vi "PLCpolling.vi"(8 "error in":errorcluster, 10 "PLC cluster":T1) -> (0 "error out":errorcluster, 1 "172.18.214.225":string[](array[string]), 2 "172.18.214.231":string[](array[string]))   [LabVIEW 2014]
uses:
  PLC-libnodave/PLC_Libnodave_wrapper_areaType.ctl
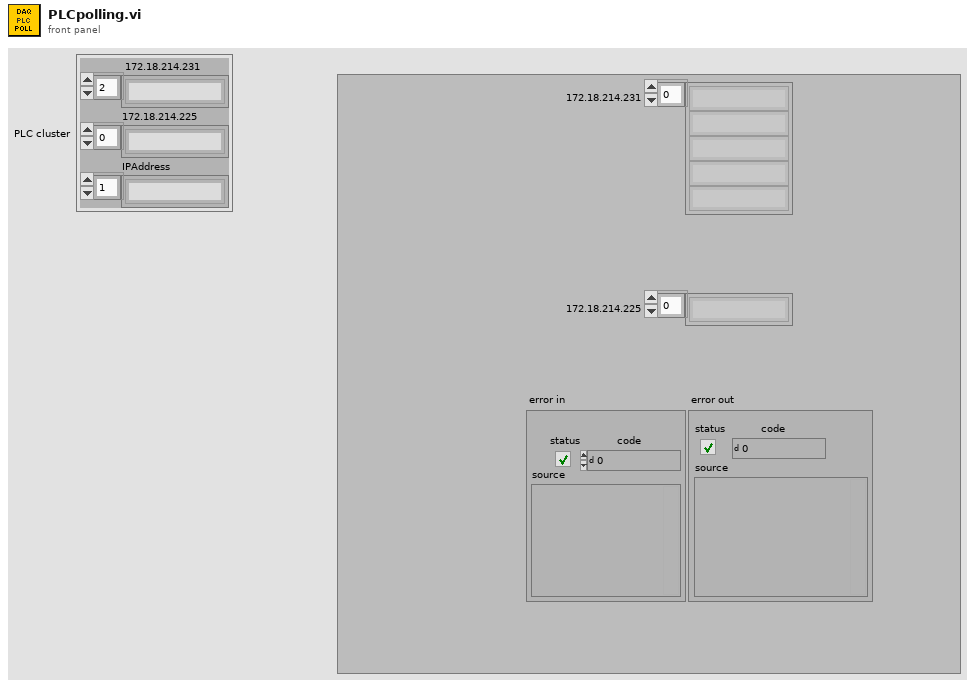
[diagram p1: front panel]
types:
  T1 = cluster{" 172.18.214.231":string[], "172.18.214.225":string[], "IPAddress":string[]}
  T2 = typedef "PLC_Libnodave_wrapper_areaType.ctl" = i32
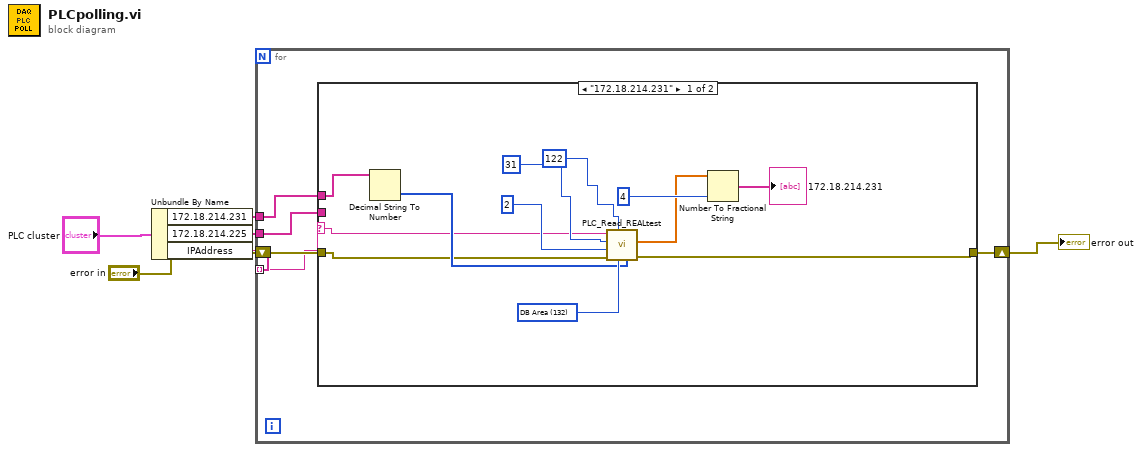
[diagram p0: block diagram]
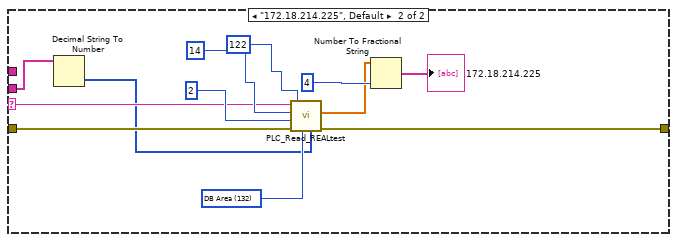
[diagram p2: hidden frame]
diagram:
  n1 = Unbundle By Name("PLC cluster") -> ("172.18.214.231"=w2:string[], "172.18.214.225"=w1:string[], "IPAddress"=w3:string[])
  n2 = for {
    shift-right: [w10] -> w5
    shift-left: "error in" -> [w11]
    tunnel: w3 -> [w9] mode=indexing
    tunnel: w2 -> [w8]
    tunnel: w1 -> [w7]
    n3 = case shown="\"172.18.214.231\"" w9 {
      selector: w9 -> [w16 w28]
      tunnel: w11 -> [w15 w31]
      tunnel: [w17 w32] -> w10
      tunnel: w8 -> [w12 _]
      tunnel: w7 -> [_ w24]
      frame "172.18.214.231" {
        w20 = T2 132 items=["P Area"=128, "I Area"=129, "O Area"=130, "M Area"=131, "DB Area"=132, "Counter Area"=40, "Timer Area"=41] ("areaType")
        n4 = Decimal String To Number(string=w12) -> (number=w18:i32[])  [unwired: 2 in, 1 out]
        n5 = call "PLC_Read_REALtest.vi"("addresses"=w18, "areaType"=w20, "cpProtocol"=122, "Error In"=w15, "slot"=2, "dataBlock"=31, "ip"=w16) -> ("Error Out"=w17:errorcluster, "results"=w14:dbl[])  [unwired: 3 in]
        n6 = Number To Fractional String(number=w14, precision (6)=i16 4) -> (F-format string=→"172.18.214.231":string[])  [unwired: 2 in]
      }
      frame "172.18.214.225", Default {
        w30 = T2 132 items=["P Area"=128, "I Area"=129, "O Area"=130, "M Area"=131, "DB Area"=132, "Counter Area"=40, "Timer Area"=41] ("areaType")
        n7 = Decimal String To Number(string=w24) -> (number=w27:i32[])  [unwired: 2 in, 1 out]
        n8 = call "PLC_Read_REALtest.vi"("addresses"=w27, "areaType"=w30, "cpProtocol"=122, "Error In"=w31, "slot"=2, "dataBlock"=14, "ip"=w28) -> ("Error Out"=w32:errorcluster, "results"=w26:dbl[])  [unwired: 3 in]
        n9 = Number To Fractional String(number=w26, precision (6)=i16 4) -> (F-format string=→"172.18.214.225":string[])  [unwired: 2 in]
      }
    }
  }
  "error out" <- w5
